vi "Measurement UI.vi"() -> ()   [LabVIEW 2021, in "Single Point_Channel Ganging.lvlib"]
uses:
  Single Point_Channel Ganging.lvlib
panel:
  in  "MeasGraphs":T1(tab)
  out "GangedCurrentGraph":waveform(dbl)[](graph) caption="AC"
  out "GangedVoltageGraph":waveform(dbl)[](graph) caption="AC"
  out "SourceCurrentGraph":waveform(dbl)[](graph) caption="AC"
  out "SourceVoltageGraph":waveform(dbl)[](graph) caption="AC"
  out "LoadCurrentGraph":waveform(dbl)[](graph) caption="AC"
  out "LoadVoltageGraph":waveform(dbl)[](graph) caption="AC"
  in  "Load slave resource names":string[](array[string])
  in  "Load master resource name":string
  in  "Source slave resource names":string[](array[string])
  in  "Source master resource name":string
  out "Ganged load currents":dbl[](array[numeric])
  out "Ganged load voltages":dbl[](array[numeric])
  out "Ganged source currents":dbl[](array[numeric])
  out "Ganged source voltages":dbl[](array[numeric])
  in  "Load source trigger":string
  out "Load currents":dbl[](array[numeric])
  out "Load voltages":dbl[](array[numeric])
  out "Source currents":dbl[](array[numeric])
  out "Source voltages":dbl[](array[numeric])
  out "dt":dbl[](array[numeric])
  in  "MeasConfigurations":T2(tab)=enum."Source Config"
  in  "Aperture time":dbl=0.01666 caption="APERTURE TIME" format="%.3ps"
  in  "Measurement time":dbl=1.0 caption="MEASUREMENT TIME" format="%.3ps"
  in  "Source ON/OFF":bool=TRUE
  in  "PPSSlaveResourceNames":refnum<k15>[](array[refnum]) caption="SLAVE RESOURCE NAMES"
  in  "PPSMasterResourceName":refnum<k15> caption="MASTER RESOURCE NAME"
  in  "Source transient response":i32(ring)=1038 caption="TRANSIENT RESPONSE" items=["Slow"=1041, "Normal"=1038, "Fast"=1039]
  in  "Source sense":i32(ring)=1009 caption="SENSE" items=["Local"=1008, "Remote"=1009]
  in  "Source voltage/current level range":dbl=20.0 caption="VOLTAGE LEVEL RANGE" format="%#_6pV"
  in  "Source voltage/current level":dbl=6.0 caption="VOLTAGE LEVEL" format="%#_6pV"
  in  "Source current/voltage limit high":dbl=25.0 caption="CURRENT LIMIT/LIMIT HIGH" format="%#_6pA"
  in  "Source current/voltage limit range":dbl=25.0 caption="CURRENT LIMIT RANGE" format="%#_6pA"
  in  "Source limit symmetry":enum32{"Symmetric", "Asymmetric"}(ring)=enum."Asymmetric" caption="LIMIT SYMMETRY"
  in  "Source current/voltage limit low":dbl=-0.6 caption="CURRENT LIMIT LOW" format="%#_6pA"
  in  "Source system configuration":enum32{"Series", "Parallel"}(ring)=enum."Parallel" caption="SYSTEM CONFIG"
  in  "Source compliance":string="Compliance"
  in  "Source sourceadapt":string="SourceAdapt"
  in  "Source output function":i32(ring)=1006 caption="OUTPUT FUNCTION" items=["DC Voltage"=1006, "DC Current"=1007]
  in  "Load sourceadapt":string="SourceAdapt"
  in  "Load trigger config":string="Trigger"
  in  "Load Source Trigger":tag caption="SOURCE TRIGGER"
  in  "Load compliance":string="Compliance"
  in  "Load system configuration":enum32{"Series", "Parallel"}(ring)=enum."Parallel" caption="SYSTEM CONFIG"
  in  "Load current/voltage limit low":dbl caption="VOLTAGE  LIMIT LOW" format="%#_6pV"
  in  "Load limit symmetry":enum32{"Symmetric", "Asymmetric"}(ring) caption="LIMIT SYMMETRY"
  in  "Load current/voltage limit range":dbl=6.0 caption="VOLTAGE LIMIT RANGE" format="%#_6pV"
  in  "Load current/voltage limit high":dbl=inf caption="VOLTAGE LIMIT/LIMIT HIGH" format="%#_6p"
  in  "Load voltage/current level":dbl=2.0 caption="CURRENT LEVEL" format="%#_6pA"
  in  "Load voltage/current level range":dbl=40.0 caption="CURRENT LEVEL RANGE" format="%#_6pA"
  in  "Load sense":i32(ring)=1009 caption="SENSE" items=["Local"=1008, "Remote"=1009]
  in  "Load transient response":i32(ring)=1038 caption="TRANSIENT RESPONSE" items=["Slow"=1041, "Normal"=1038, "Fast"=1039]
  in  "Load output function":i32(ring)=1007 caption="OUTPUT FUNCTION" items=["DC Voltage"=1006, "DC Current"=1007]
  in  "Load ON/OFF":bool=TRUE
  in  "LoadMasterResourceName":refnum<k15> caption="MASTER RESOURCE NAME"
  in  "LoadSlaveResourceNames":refnum<k15>[](array[refnum]) caption="SLAVE RESOURCE NAMES"
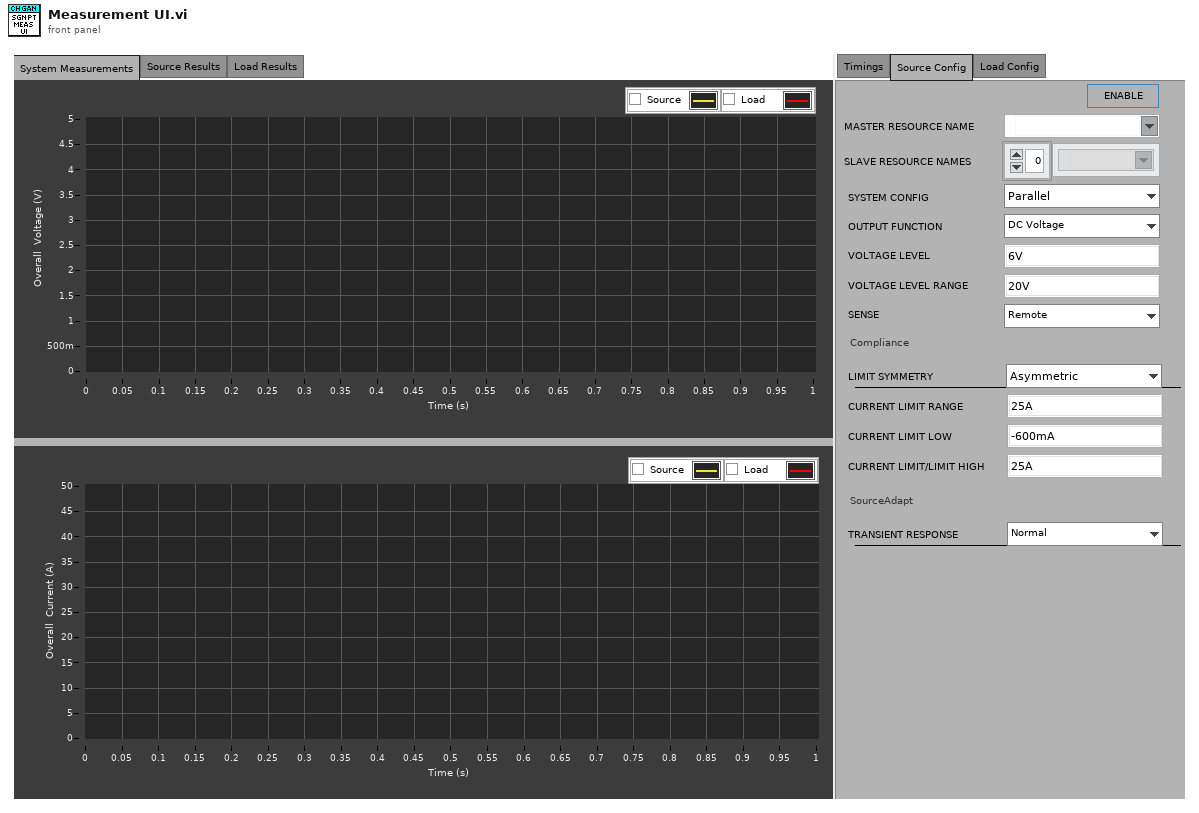
[diagram p1: front panel]
types:
  T1 = enum32{"System Measurements", "Source Results", "Load Results", "Hidden Controls"}
  T2 = enum32{"Timings", "Source Config", "Load Config"}
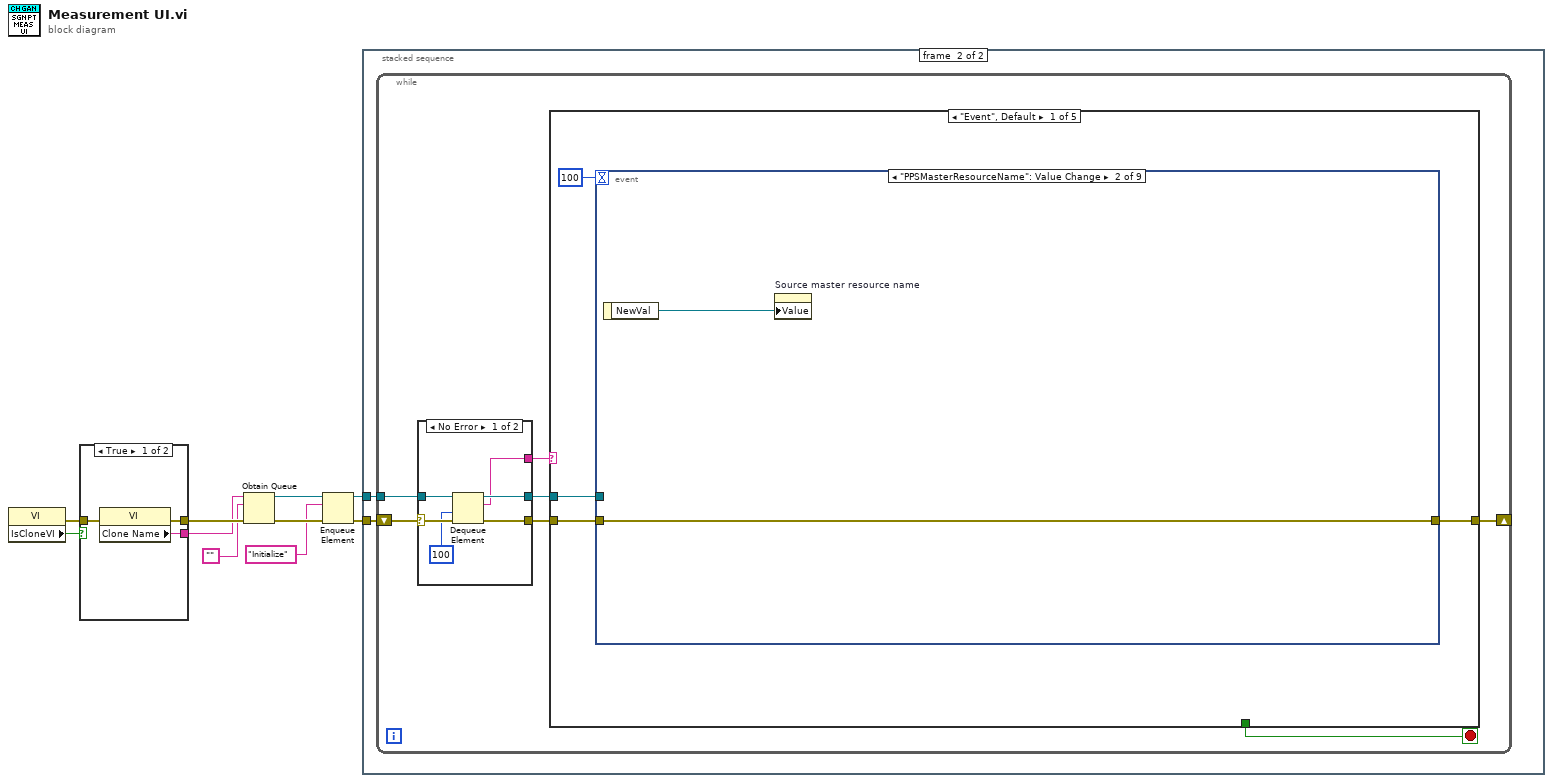
[diagram p0: block diagram]
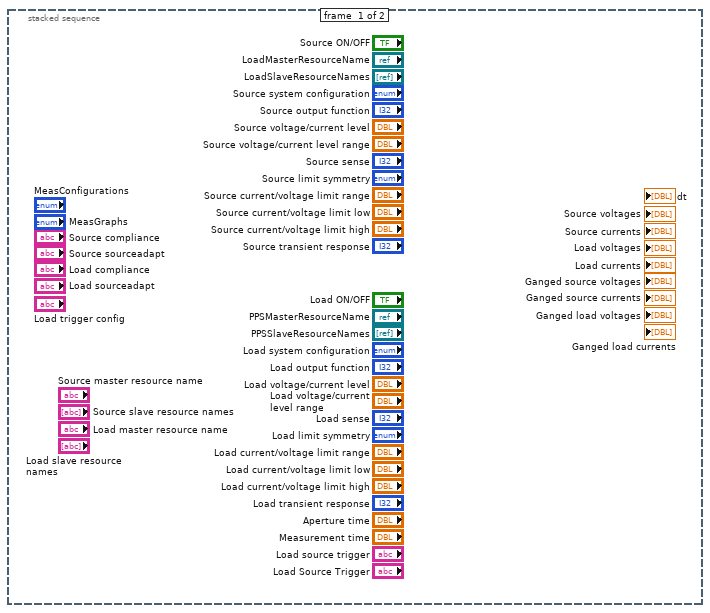
[diagram p2: hidden frame]
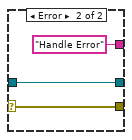
[diagram p3: hidden frame]
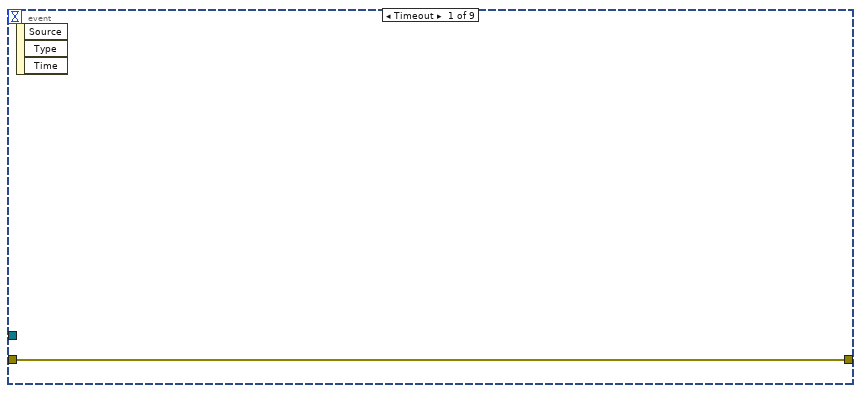
[diagram p4: hidden frame]
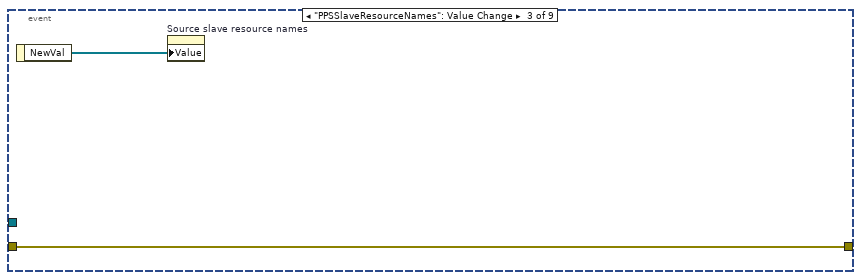
[diagram p5: hidden frame]
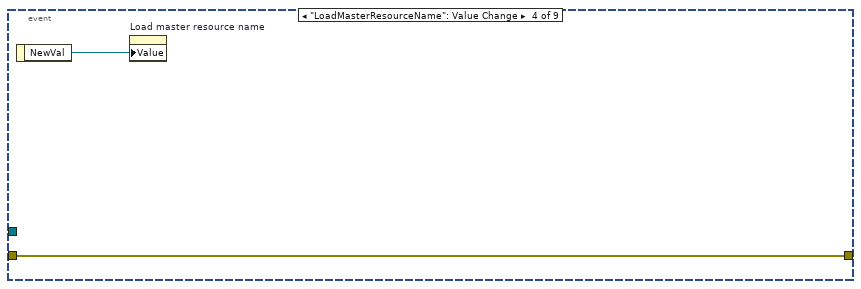
[diagram p6: hidden frame]
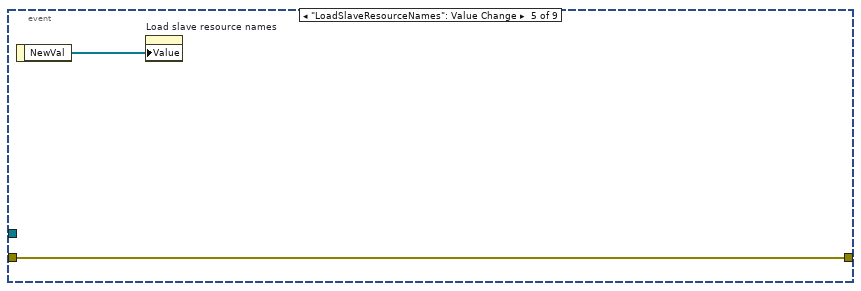
[diagram p7: hidden frame]
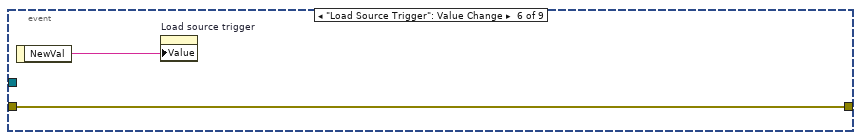
[diagram p8: hidden frame]
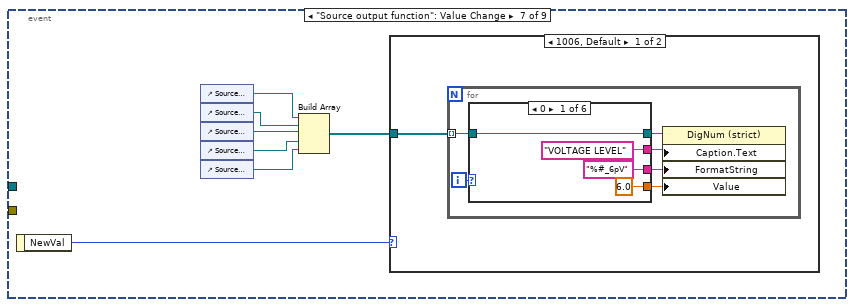
[diagram p9: hidden frame]
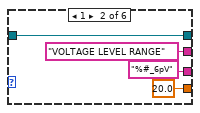
[diagram p10: hidden frame]
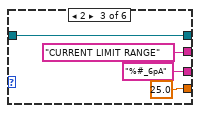
[diagram p11: hidden frame]
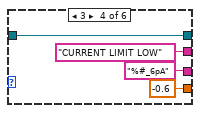
[diagram p12: hidden frame]
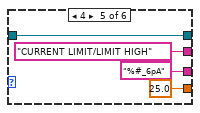
[diagram p13: hidden frame]
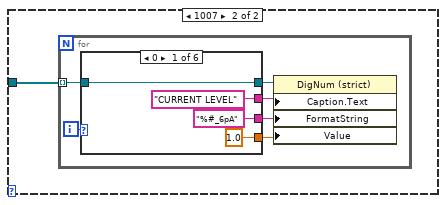
[diagram p15: hidden frame]
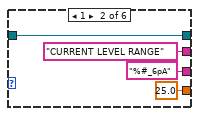
[diagram p16: hidden frame]
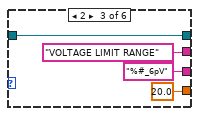
[diagram p17: hidden frame]
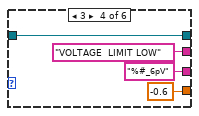
[diagram p18: hidden frame]
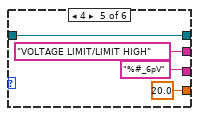
[diagram p19: hidden frame]
diagram:
  n1 = property class="VI"() -> (error out=w1:errorcluster, "IsCloneVI"=w2:bool)  [unwired: 2 in, 1 out]
  n2 = case shown="True" w2 {
    tunnel: [w13 w16] -> w10
    tunnel: [w12 w15] -> w9
    tunnel: w1 -> [w11 w14]
    frame True {
      n3 = property class="VI"(error in=w11) -> (error out=w13:errorcluster, "Clone Name"=w12:string)  [unwired: 1 in, 1 out]
    }
    frame False {
      n4 = property class="VI"(error in=w14) -> (error out=w16:errorcluster, "Name"=w15:string)  [unwired: 1 in, 1 out]
    }
  }
  n5 = Obtain Queue(name (unnamed)=w9, element data type="", error in (no error)=w10) -> (queue out=w6:refnum<queue>, error out=w8:errorcluster)  [unwired: 2 in, 1 out]
  n6 = Enqueue Element(queue=w6, element="Initialize", error in (no error)=w8) -> (queue out=w5:refnum<queue>, error out=w7:errorcluster)  [unwired: 1 in, 1 out]
  n7 = stacked-sequence {
    tunnel: w7 -> [_ w18]
    tunnel: w5 -> [_ w17]
    frame #0 {
    }
    frame #1 {
      n8 = while {
        shift-right: [w20] -> _
        shift-left: w18 -> [w25]
        tunnel: w17 -> [w23]
        stop <- w19 stop-if-true
        n9 = case shown="No Error" w25 {
          selector: w25 -> [w31 w34]
          tunnel: [w30 w34] -> w24
          tunnel: w23 -> [w29 w33]
          tunnel: [w28 w33] -> w22
          tunnel: [w27 "Handle Error"] -> w21
          frame No Error {
            n10 = Dequeue Element(queue=w29, timeout in ms (-1)=100, error in (no error)=w31) -> (queue out=w28:refnum<queue>, element=w27:string, error out=w30:errorcluster)  [unwired: 1 out]
          }
          frame Error {
          }
        }
        n11 = case shown="\"Event\", Default" w21 {
          tunnel: w24 -> [w37 w178 w209 w241 w242]
          tunnel: w22 -> [w35 _ _ w239 _]
          tunnel: [w38 w178 w209 w236 w242] -> w20
          tunnel: [_ _ _ TRUE _] -> w19
          frame "Event", Default {
            n12 = event shown="[1] \"PPSMasterResourceName\": Value Change" {
              selector: _ -> [_ _ _ _ _ _ _ _ _]
              dyn-events: _ -> [_ _ _ _ _ _ _ _ _]
              timeout: 100 -> [_ _ _ _ _ _ _ _ _]
              tunnel: [w39 w41 w43 w44 w46 w48 _ _ w175] -> w38
              tunnel: w37 -> [w39 w41 w43 w44 w46 w48 _ _ w176]
              tunnel: w35 -> [_ _ _ _ _ _ _ _ w174]
              event Timeout {
                n13 = event-data() -> ()  [unwired: 1 in, 3 out]
              }
              event "PPSMasterResourceName": Value Change {
                n14 = event-data() -> ("NewVal"=w40:refnum<k15>)  [unwired: 1 in]
                n15 = property on="Source master resource name" class="Str"("Value"=w40) -> ()  [unwired: 2 in, 2 out]
              }
              event "PPSSlaveResourceNames": Value Change {
                n16 = event-data() -> ("NewVal"=w42:refnum<k15>[])  [unwired: 1 in]
                n17 = property on="Source slave resource names" class="Arr (strict)"("Value"=w42) -> ()  [unwired: 2 in, 2 out]
              }
              event "LoadMasterResourceName": Value Change {
                n18 = event-data() -> ("NewVal"=w45:refnum<k15>)  [unwired: 1 in]
                n19 = property on="Load master resource name" class="Str"("Value"=w45) -> ()  [unwired: 2 in, 2 out]
              }
              event "LoadSlaveResourceNames": Value Change {
                n20 = event-data() -> ("NewVal"=w47:refnum<k15>[])  [unwired: 1 in]
                n21 = property on="Load slave resource names" class="Arr (strict)"("Value"=w47) -> ()  [unwired: 2 in, 2 out]
              }
              event "Load Source Trigger": Value Change {
                n22 = event-data() -> ("NewVal"=w49:tag)  [unwired: 1 in]
                n23 = property on="Load source trigger" class="Str"("Value"=w49) -> ()  [unwired: 2 in, 2 out]
              }
              event "Source output function": Value Change {
                n24 = event-data() -> ("NewVal"=w56:i32)  [unwired: 1 in]
                n25 = control-ref of="Source voltage/current level"() -> (w55:refnum<vi>)
                n26 = control-ref of="Source voltage/current level range"() -> (w54:refnum<vi>)
                n27 = control-ref of="Source current/voltage limit range"() -> (w53:refnum<vi>)
                n28 = control-ref of="Source current/voltage limit low"() -> (w52:refnum<vi>)
                n29 = control-ref of="Source current/voltage limit high"() -> (w51:refnum<vi>)
                n30 = Build Array(w55, w54, w53, w52, w51) -> (w50:refnum<vi>[])
                n31 = case shown="1006, Default" w56 {
                  tunnel: w50 -> [w57 w84]
                  frame 1006, Default {
                    n32 = for {
                      tunnel: w57 -> [w61] mode=indexing
                      i -> [w63]
                      n33 = case shown="0" w63 {
                        tunnel: [w67 w71 w75 w78 w82 _] -> w62
                        tunnel: w61 -> [w67 w71 w75 w78 w82 _]
                        tunnel: ["VOLTAGE LEVEL" ("Caption.Text") "VOLTAGE LEVEL RANGE" ("Caption.Text") "CURRENT LIMIT RANGE" ("Caption.Text") "CURRENT LIMIT LOW" ("Caption.Text") "CURRENT LIMIT/LIMIT HIGH" ("Caption.Text") _] -> w60
                        tunnel: ["%#_6pV" ("Format String") "%#_6pV" ("Format String") "%#_6pA" ("Format String") "%#_6pA" ("Format String") "%#_6pA" ("Format String") _] -> w59
                        tunnel: [6.0 ("Value") 20.0 ("Value") 25.0 ("Value") -0.6 ("Value") 25.0 ("Value") _] -> w58
                        frame 0 {
                        }
                        frame 1 {
                        }
                        frame 2 {
                        }
                        frame 3 {
                        }
                        frame 4 {
                        }
                        frame Default {
                        }
                      }
                      n34 = property class="DigNum (strict)"(reference=w62, "Caption.Text"=w60, "FormatString"=w59, "Value"=w58) -> ()  [unwired: 1 in, 2 out]
                    }
                  }
                  frame 1007 {
                    n35 = for {
                      tunnel: w84 -> [w88] mode=indexing
                      i -> [w90]
                      n36 = case shown="0" w90 {
                        tunnel: [w94 w98 w102 w105 w109 _] -> w89
                        tunnel: w88 -> [w94 w98 w102 w105 w109 _]
                        tunnel: ["CURRENT LEVEL" ("Caption.Text") "CURRENT LEVEL RANGE" ("Caption.Text") "VOLTAGE LIMIT RANGE" ("Caption.Text") "VOLTAGE  LIMIT LOW" ("Caption.Text") "VOLTAGE LIMIT/LIMIT HIGH" ("Caption.Text") _] -> w87
                        tunnel: ["%#_6pA" ("Format String") "%#_6pA" ("Format String") "%#_6pV" ("Format String") "%#_6pV" ("Format String") "%#_6pV" ("Format String") _] -> w86
                        tunnel: [1.0 ("Value") 25.0 ("Value") 20.0 ("Value") -0.6 ("Value") 20.0 ("Value") _] -> w85
                        frame 0 {
                        }
                        frame 1 {
                        }
                        frame 2 {
                        }
                        frame 3 {
                        }
                        frame 4 {
                        }
                        frame Default {
                        }
                      }
                      n37 = property class="DigNum (strict)"(reference=w89, "Caption.Text"=w87, "FormatString"=w86, "Value"=w85) -> ()  [unwired: 1 in, 2 out]
                    }
                  }
                }
              }
              event "Load output function": Value Change {
                n38 = event-data() -> ("NewVal"=w112:i32)  [unwired: 1 in]
                n39 = control-ref of="Load voltage/current level"() -> (w117:refnum<vi>)
                n40 = control-ref of="Load voltage/current level range"() -> (w116:refnum<vi>)
                n41 = control-ref of="Load current/voltage limit range"() -> (w115:refnum<vi>)
                n42 = control-ref of="Load current/voltage limit low"() -> (w114:refnum<vi>)
                n43 = control-ref of="Load current/voltage limit high"() -> (w113:refnum<vi>)
                n44 = Build Array(w117, w116, w115, w114, w113) -> (w111:refnum<vi>[])
                n45 = case shown="1007, Default" w112 {
                  tunnel: w111 -> [w118 w145]
                  frame 1006 {
                    n46 = for {
                      tunnel: w118 -> [w122] mode=indexing
                      i -> [w124]
                      n47 = case shown="0" w124 {
                        tunnel: [w128 w132 w136 w139 w143 _] -> w123
                        tunnel: w122 -> [w128 w132 w136 w139 w143 _]
                        tunnel: ["VOLTAGE LEVEL" ("Caption.Text") "VOLTAGE LEVEL RANGE" ("Caption.Text") "CURRENT LIMIT RANGE" ("Caption.Text") "CURRENT LIMIT LOW" ("Caption.Text") "CURRENT LIMIT/LIMIT HIGH" ("Caption.Text") _] -> w121
                        tunnel: ["%#_6pV" ("Format String") "%#_6pV" ("Format String") "%#_6pA" ("Format String") "%#_6pA" ("Format String") "%#_6pA" ("Format String") _] -> w120
                        tunnel: [3.3 ("Value") 6.0 ("Value") 40.0 ("Value") 0.0 ("Value") 40.0 ("Value") _] -> w119
                        frame 0 {
                        }
                        frame 1 {
                        }
                        frame 2 {
                        }
                        frame 3 {
                        }
                        frame 4 {
                        }
                        frame Default {
                        }
                      }
                      n48 = property class="DigNum (strict)"(reference=w123, "Caption.Text"=w121, "FormatString"=w120, "Value"=w119) -> ()  [unwired: 1 in, 2 out]
                    }
                  }
                  frame 1007, Default {
                    n49 = for {
                      tunnel: w145 -> [w149] mode=indexing
                      i -> [w151]
                      n50 = case shown="0" w151 {
                        tunnel: [w155 w159 w163 w166 w171 _] -> w150
                        tunnel: w149 -> [w155 w159 w163 w166 w171 _]
                        tunnel: ["CURRENT LEVEL" ("Caption.Text") "CURRENT LEVEL RANGE" ("Caption.Text") "VOLTAGE LIMIT RANGE" ("Caption.Text") "VOLTAGE  LIMIT LOW" ("Caption.Text") "VOLTAGE LIMIT/LIMIT HIGH" ("Caption.Text") _] -> w148
                        tunnel: ["%#_6pA" ("Format String") "%#_6pA" ("Format String") "%#_6pV" ("Format String") "%#_6pV" ("Format String") "%#_6p" ("Format String") _] -> w147
                        tunnel: [2.0 ("Value") 40.0 ("Value") 6.0 ("Value") 0.0 ("Value") w169 _] -> w146
                        frame 0 {
                        }
                        frame 1 {
                        }
                        frame 2 {
                        }
                        frame 3 {
                        }
                        frame 4 {
                          n51 = Reciprocal(x=0.0) -> (1/x=w169:dbl)
                        }
                        frame Default {
                        }
                      }
                      n52 = property class="DigNum (strict)"(reference=w150, "Caption.Text"=w148, "FormatString"=w147, "Value"=w146) -> ()  [unwired: 1 in, 2 out]
                    }
                  }
                }
              }
              event Panel Close? {
                n53 = event-data() -> ()  [unwired: 1 in, 4 out]
                n54 = Enqueue Element(queue=w174, element="Exit", error in (no error)=w176) -> (error out=w175:errorcluster)  [unwired: 1 in, 2 out]
                n55 = event-data("Discard?"=TRUE) -> ()  [unwired: 1 in, 1 out]
              }
            }
          }
          frame "Initialize" {
          }
          frame "Post UI Update" {
            # "This case will be triggered, after framework updates the User interface with result values."
            n56 = local read "Source voltages"() -> (w196:dbl[])
            n57 = local read "Source currents"() -> (w199:dbl[])
            n58 = local read "Load voltages"() -> (w198:dbl[])
            n59 = local read "Load currents"() -> (w197:dbl[])
            n60 = local read "Ganged source voltages"() -> (w191:dbl[])
            n61 = local read "Ganged source currents"() -> (w181:dbl[])
            n62 = local read "Ganged load voltages"() -> (w189:dbl[])
            n63 = local read "Ganged load currents"() -> (w180:dbl[])
            n64 = local read "dt"() -> (w188:dbl[])
            n65 = Array Size(array=w188) -> (size(s)=w203:i32)
            n66 = Array Size(array=w196) -> (size(s)=w205:i32)
            n67 = Array Size(array=w199) -> (size(s)=w204:i32)
            n68 = Array Size(array=w198) -> (size(s)=w207:i32)
            n69 = Array Size(array=w197) -> (size(s)=w208:i32)
            n70 = Index Array(array=w188, index=0) -> (element=w182:dbl)
            n71 = Divide(x=w205, y=w203) -> (x/y=w206:dbl)
            n72 = Divide(x=w208, y=w203) -> (x/y=w202:dbl)
            n73 = Divide(x=w207, y=w203) -> (x/y=w201:dbl)
            n74 = Divide(x=w204, y=w203) -> (x/y=w200:dbl)
            n75 = Bundle By Name("dt"=w182, "Y"=w191) -> (w190:waveform(dbl))  [unwired: 1 in]
            n76 = Bundle By Name("dt"=w182, "Y"=w189) -> (w186:waveform(dbl))  [unwired: 1 in]
            n77 = Bundle By Name("dt"=w182, "Y"=w181) -> (w183:waveform(dbl))  [unwired: 1 in]
            n78 = Bundle By Name("dt"=w182, "Y"=w180) -> (w184:waveform(dbl))  [unwired: 1 in]
            n79 = for {
              N: w203 -> [_]
              tunnel: w206 -> [w232]
              shift-right: [w233] -> _
              shift-left: w196 -> [w234]
              tunnel: [w227] -> w195 mode=indexing
              tunnel: [w226] -> w194 mode=indexing
              tunnel: [w225] -> w193 mode=indexing
              tunnel: [w224] -> w192 mode=indexing
              shift-right: [w218] -> _
              shift-left: w199 -> [w219]
              shift-right: [w216] -> _
              shift-left: w198 -> [w217]
              shift-right: [w214] -> _
              shift-left: w197 -> [w215]
              tunnel: w202 -> [w213]
              tunnel: w201 -> [w212]
              tunnel: w200 -> [w211]
              tunnel: w188 -> [w210] mode=indexing
              n80 = Delete From Array(array=w234, length=w232, index=0) -> (deleted portion=w223:dbl[], array with subset deleted=w233:dbl[])
              n81 = Delete From Array(array=w219, length=w211, index=0) -> (deleted portion=w222:dbl[], array with subset deleted=w218:dbl[])
              n82 = Delete From Array(array=w217, length=w212, index=0) -> (deleted portion=w221:dbl[], array with subset deleted=w216:dbl[])
              n83 = Delete From Array(array=w215, length=w213, index=0) -> (deleted portion=w220:dbl[], array with subset deleted=w214:dbl[])
              n84 = Bundle By Name("dt"=w210, "Y"=w223) -> (w227:waveform(dbl))  [unwired: 1 in]
              n85 = Bundle By Name("dt"=w210, "Y"=w222) -> (w226:waveform(dbl))  [unwired: 1 in]
              n86 = Bundle By Name("dt"=w210, "Y"=w221) -> (w225:waveform(dbl))  [unwired: 1 in]
              n87 = Bundle By Name("dt"=w210, "Y"=w220) -> (w224:waveform(dbl))  [unwired: 1 in]
            }
            "SourceVoltageGraph" <- w195
            "SourceCurrentGraph" <- w194
            "LoadVoltageGraph" <- w193
            "LoadCurrentGraph" <- w192
            n88 = Build Array(w190, w186) -> (→"GangedVoltageGraph":waveform(dbl)[])
            n89 = Build Array(w183, w184) -> (→"GangedCurrentGraph":waveform(dbl)[])
          }
          frame "Exit" {
            # "This case is triggered to close the User Interface from framework"
            n90 = Flush Queue(queue=w239, error in (no error)=w241) -> (queue out=w238:refnum<queue>, error out=w237:errorcluster)  [unwired: 1 out]
            n91 = Release Queue(queue=w238, force destroy? (F)=TRUE, error in (no error)=w237) -> (error out=w236:errorcluster)  [unwired: 2 out]
          }
          frame "Handle Error" {
          }
        }
      }
    }
  }
